vi "任意时刻单点闹钟.vi"(8 "Error In":errorcluster caption="错误输入", 10 "偏移量（秒）":dbl, 11 "定闹时刻":timestamp) -> (0 "Error Out":errorcluster caption="错误输出", 2 "离定闹时间还有（秒）":dbl, 3 "时间到":bool)   [LabVIEW 2012]
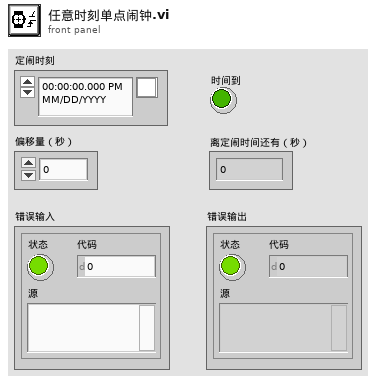
[diagram p1: front panel]
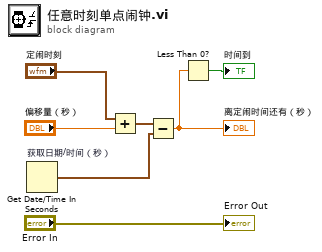
[diagram p0: block diagram]
diagram:
  n1 = Get Date/Time In Seconds "获取日期/时间（秒）"() -> (seconds since 1Jan1904=w4:timestamp)
  n2 = Add(x="定闹时刻", y="偏移量（秒）") -> (x+y=w3:timestamp)
  n3 = Subtract(x=w3, y=w4) -> (x-y=w1:dbl)
  "离定闹时间还有（秒）" <- w1
  n4 = Less Than 0?(x=w1) -> (x < 0?=→"时间到":bool)
  "Error Out" <- "Error In"
